vi "LOGOUT.vi"() -> ()   [LabVIEW 2017]
uses:
  GLOBAL/auto.vi
panel:
  out "error out":errorcluster
  in  "error in":errorcluster
  # "LOGOUT"
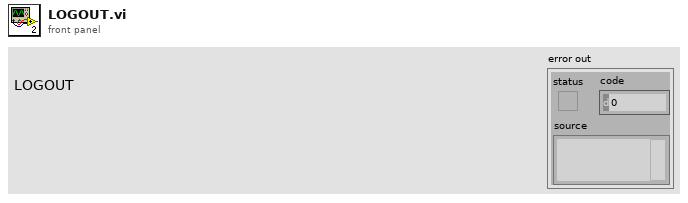
[diagram p1: front panel]
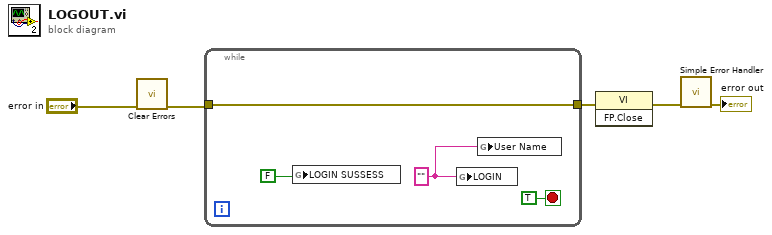
[diagram p0: block diagram]
diagram:
  n1 = call <vilib>:"Clear Errors.vi"("error in (no error)"="error in") -> ("error out"=w4:errorcluster)  [unwired: 5 in, 1 out]
  n2 = while {
    tunnel: [w8] -> w5
    tunnel: w4 -> [w8]
    stop <- TRUE stop-if-true
    w7 = "" ("f")
    n3 = global write "auto.vi" "LOGIN SUSSESS"(FALSE) -> ()
    n4 = global write "auto.vi" "LOGIN"(w7) -> ()
    n5 = global write "auto.vi" "User Name"(w7) -> ()
  }
  n6 = invoke class="VI" method="FP.Close"(error in=w5) -> (error out=w2:errorcluster)  [unwired: 2 in, 2 out]
  n7 = call <vilib>:"Simple Error Handler.vi"("error in (no error)"=w2) -> ("error out"=→"error out":errorcluster)  [unwired: 4 in, 4 out]
